vi "Set_Volume_and_Rate.vi"(8 "error in (no error)":errorcluster, 9 "Volume (100)":i32=100, 10 "Speech Rate (0)":i32, 11 "speech_voce_refs (in)":T1) -> (0 "error out":errorcluster, 3 "speech object references (out)":T1)   [LabVIEW 8.6]
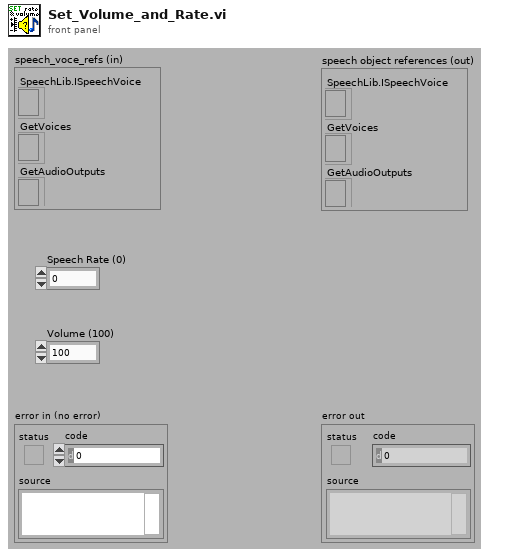
[diagram p1: front panel]
types:
  T1 = cluster{"SpeechLib.ISpeechVoice":refnum<k7>, "GetVoices":refnum<k7>, "GetAudioOutputs":refnum<k7>}
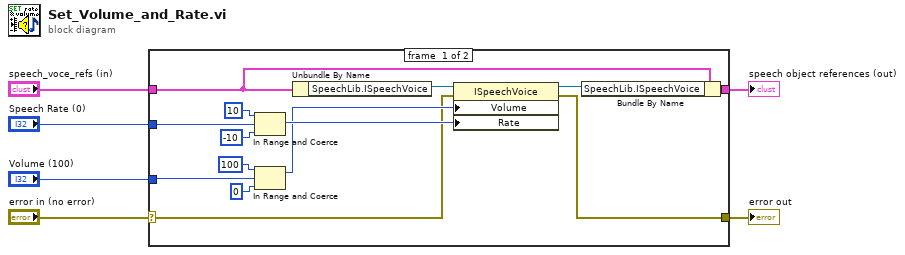
[diagram p0: block diagram]
diagram:
  n1 = case shown="No Error" "error in (no error)" {
    selector: "error in (no error)" -> [w7 w22]
    tunnel: "speech_voce_refs (in)" -> [w19 w21]
    tunnel: [w17 w21] -> w5
    tunnel: [w16 w22] -> w4
    tunnel: "Speech Rate (0)" -> [w15 _]
    tunnel: "Volume (100)" -> [w11 _]
    frame #0 {
      n2 = In Range and Coerce(upper limit=10, x=w15, lower limit=-10) -> (coerced(x)=w12:i32)  [unwired: 1 out]
      n3 = In Range and Coerce(upper limit=100, x=w11, lower limit=0) -> (coerced(x)=w8:i32)  [unwired: 1 out]
      n4 = Unbundle By Name(w19) -> ("SpeechLib.ISpeechVoice"=w20:refnum<k7>)
      n5 = property class="ISpeechVoice"(reference=w20, error in=w7, "Volume"=w8, "Rate"=w12) -> (reference out=w18:refnum<k7>, error out=w16:errorcluster)
      n6 = Bundle By Name(cluster=w19, "SpeechLib.ISpeechVoice"=w18) -> (w17:T1)
    }
    frame #1 {
    }
  }
  "error out" <- w4
  "speech object references (out)" <- w5
